vi "Begin.vi"(8 "error in":errorcluster) -> (0 "error out":errorcluster)   [LabVIEW 2015]
doc: "Called before other user functions, this VI is expected to open initial I/O refnums, load in file data, and do all program initialization. Notice that the <B>error out</B> terminal is simply used for data flow. Wiring it to other structures or subVIs ensures that this VI runs first."
uses:
  <vilib>/Rock Robotics/WPI/DriverStation/WPI_DriverStationRobotMode2.ctl
  <vilib>/Rock Robotics/WPI/Joystick/WPI_JoystickDeviceEnum.ctl
  <vilib>/Rock Robotics/SystemInterfaces/DIO/FPGA_DIOPWMChannel.ctl
  Robot Global Data.vi
  <vilib>/Rock Robotics/Network Tables/NT Write String Array.vi
  <vilib>/Rock Robotics/WPI/MotorControl/WPI_MotorControlOpen Talon.vi
  <vilib>/Rock Robotics/WPI/MotorControl/WPI_MotorControlOpen Victor.vi
  <vilib>/Rock Robotics/WPI/RobotDrive/WPI_RobotDriveOpen4MotorWithTalon.vi
  SubSystems/References/Refnums.vi
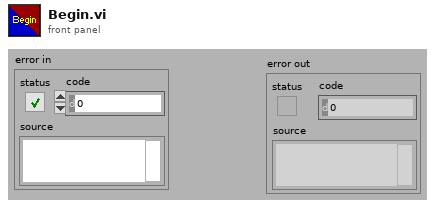
[diagram p1: front panel]
types:
  T1 = typedef "FPGA_DIOPWMChannel.ctl" = enum8{"PWM 0", "PWM 1", "PWM 2", "PWM 3", "PWM 4", "PWM 5", "PWM 6", "PWM 7", "PWM 8", "PWM 9", "PWM MXP 0", "PWM MXP 1", "PWM MXP 2", "PWM MXP 3", "PWM MXP 4", "PWM MXP 5", "PWM MXP 6", "PWM MXP 7", "PWM MXP 8", "PWM MXP 9", "Invalid"}
  T2 = typedef "WPI_JoystickDeviceEnum.ctl" = enum16{"USB 0", "USB 1", "USB 2", "USB 3", "USB 4", "USB 5"}
  T3 = typedef "WPI_DriverStationRobotMode2.ctl" = enum16{"Autonomous Disabled", "Autonomous Enabled", "Teleop Disabled", "Teleop Enabled", "Disconnected", "Finish", "Test Disabled", "Test Enabled", "Emergency Stopped"}
  T4 = typedef "WPI_JoystickDevRef.ctl" = cluster{"Device":T2}
  T5 = typedef "WPI_MotorControlDeviceRef.ctl" = cluster{"DeviceStatus":errorcluster, "Type":T6, "PWM":cluster{"PWM Channel":T1, "DeadBand":T7}, "CAN":cluster{"Device Number":u8, "Control Mode":T8, "Semaphore":T9, "Max Vout":dbl, "TalonSRX Control Mode":T10}, "Invert":bool}
  T6 = typedef "WPI_MotorControlType.ctl" = enum16{"PWM", "CAN", "CANTalonSRX"}
  T7 = typedef "WPI_PWMDeadband.ctl" = cluster{"Name":string, "maxPositivePwm":i32, "minPositivePwm":i32, "centerPwm":i32, "maxNegativePwm":i32, "minNegativePwm":i32, "angularRange":u16}
  T8 = typedef "WPI_CANJaguar_ControlMode.ctl" = enum8{"Percent VBus", "Current", "Speed", "Position", "Voltage"}
  T9 = typedef "Semaphore RefNum" = refnum<k1>
  T10 = typedef "WPI_CANTalonSRX_APIControlMode.ctl" = enum8{"Percent VBus", "Speed", "Position", "Slave", "Unchanged / Invalid", "Voltage Compensation", "Current", "Motion Profile"}
  T11 = typedef "WPI_RobotDriveDevRef.ctl" = cluster{"DevStatus":errorcluster, "Motors[]":T5[], "Square Inputs":bool, "Max Output":dbl}
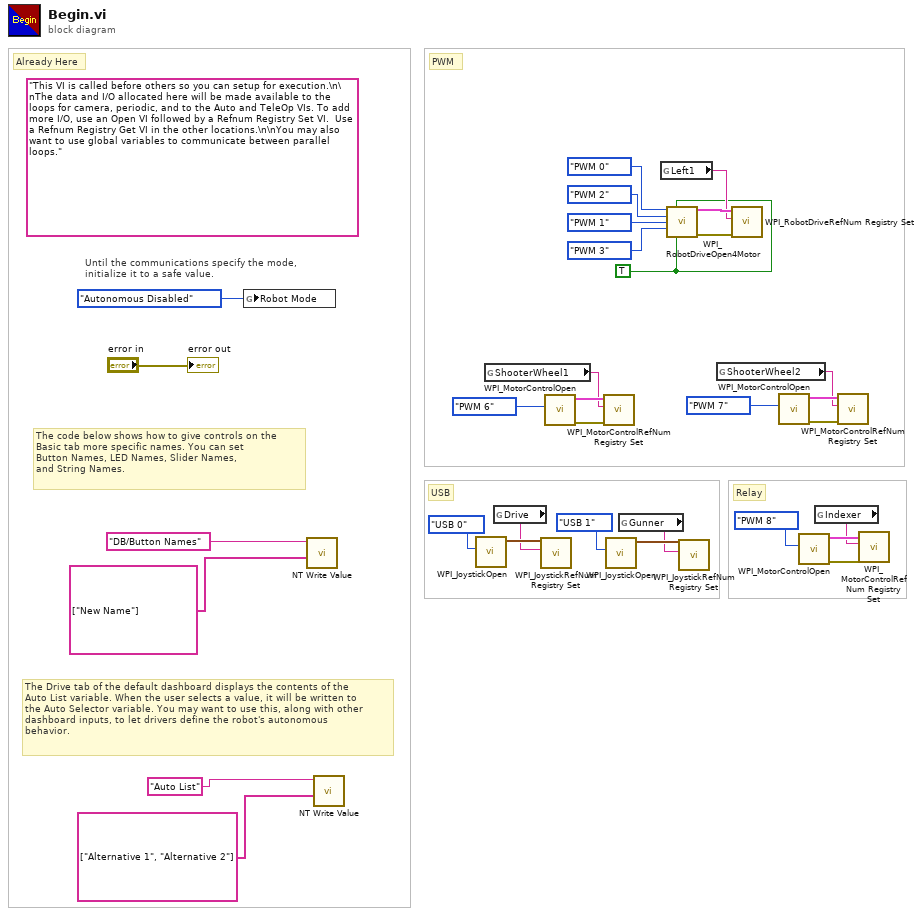
[diagram p0: block diagram]
diagram:
  w5 = TRUE ("Left Motor Inverted")
  (unwired) "This VI is called before others so you can setup for execution.\n\nThe data and I/O allocated here will be made available to the loops for camera, periodic, and to the Auto and TeleOp VIs. To add more I/O, use an Open VI followed by a Refnum Registry Set VI.  Use a Refnum Registry Get VI in the other locations.\n\nYou may also want to use global variables to communicate between parallel loops."
  # "PWM"
  # "Already Here"
  # "USB"
  # "Relay"
  # "The Drive tab of the default dashboard displays the contents of the\nAuto List variable. When the user selects a value, it will be written to\nthe Auto Selector variable. You may want to use this, along with other\ndashboard inputs, to let drivers define the robot's autonomous\nbehavior."
  # "The code below shows how to give controls on the\nBasic tab more specific names. You can set\nButton Names, LED Names, Slider Names,\nand String Names."
  # "Until the communications specify the mode,\ninitialize it to a safe value."
  n1 = global write "Robot Global Data.vi" "Robot Mode"(WPI_DriverStationRobotMode2."Autonomous Disabled" ("Robot Mode")) -> ()
  n2 = call-poly <vilib>:"NT Write Value.vi"("String Array"=string[] ["New Name"], "Name"="DB/Button Names") -> ()  [unwired: 9 in, 1 out]
  n3 = call-poly <vilib>:"NT Write Value.vi"("String Array"=string[] ["Alternative 1", "Alternative 2"], "Name"="Auto List") -> ()  [unwired: 9 in, 1 out]
  n4 = call <vilib>:"WPI_JoystickOpen.vi"("JoystickDevice"=WPI_JoystickDeviceEnum."USB 0") -> ("JoystickDevRef"=w26:T4)  [unwired: 10 in]
  n5 = global read "Refnums.vi" "ShooterWheel1"() -> (w13:string)
  n6 = global read "Refnums.vi" "Drive"() -> (w24:string)
  n7 = call <vilib>:"WPI_JoystickRefNum Registry Set.vi"("refnum name"=w24, "JoystickDevRef"=w26) -> ()  [unwired: 8 in, 2 out]
  n8 = call-poly <vilib>:"WPI_MotorControlOpen.vi"("PWM Channel"=FPGA_DIOPWMChannel."PWM 6") -> ("error out"=w15:errorcluster, "MotorControlDeviceRef"=w14:T5)  [unwired: 9 in]
  n9 = call <vilib>:"WPI_MotorControlRefNum Registry Set.vi"("error in (no error)"=w15, "refnum name"=w13, "MotorControlDevRef"=w14) -> ()  [unwired: 7 in, 2 out]
  n10 = call <vilib>:"WPI_JoystickOpen.vi"("JoystickDevice"=WPI_JoystickDeviceEnum."USB 1") -> ("JoystickDevRef"=w25:T4)  [unwired: 10 in]
  n11 = global read "Refnums.vi" "Gunner"() -> (w23:string)
  n12 = global read "Refnums.vi" "Left1"() -> (w6:string)
  n13 = call-poly <vilib>:"WPI_RobotDriveOpen4Motor.vi"("Rear Left Motor"=FPGA_DIOPWMChannel."PWM 0" ("Right Motor"), "Rear Left Motor Inverted"=w5, "Rear Right Motor"=FPGA_DIOPWMChannel."PWM 2" ("Left Motor"), "Front Left Motor"=FPGA_DIOPWMChannel."PWM 1" ("Left Motor"), "Front Right Motor"=FPGA_DIOPWMChannel."PWM 3" ("Left Motor"), "Front Left Motor Inverted"=w5) -> ("RobotDriveDevRef"=w8:T11, "error out"=w7:errorcluster)  [unwired: 8 in]
  n14 = call <vilib>:"WPI_JoystickRefNum Registry Set.vi"("refnum name"=w23, "JoystickDevRef"=w25) -> ()  [unwired: 8 in, 2 out]
  n15 = global read "Refnums.vi" "ShooterWheel2"() -> (w16:string)
  n16 = call <vilib>:"WPI_RobotDriveRefNum Registry Set.vi"("error in (no error)"=w7, "refnum name"=w6, "RobotDriveDevRef"=w8) -> ()  [unwired: 7 in, 2 out]
  n17 = call-poly <vilib>:"WPI_MotorControlOpen.vi"("PWM Channel"=FPGA_DIOPWMChannel."PWM 7") -> ("error out"=w18:errorcluster, "MotorControlDeviceRef"=w17:T5)  [unwired: 9 in]
  n18 = call-poly <vilib>:"WPI_MotorControlOpen.vi"("PWM Channel"=FPGA_DIOPWMChannel."PWM 8") -> ("error out"=w11:errorcluster, "MotorControlDeviceRef"=w10:T5)  [unwired: 9 in]
  n19 = global read "Refnums.vi" "Indexer"() -> (w9:string)
  n20 = call <vilib>:"WPI_MotorControlRefNum Registry Set.vi"("error in (no error)"=w18, "refnum name"=w16, "MotorControlDevRef"=w17) -> ()  [unwired: 7 in, 2 out]
  n21 = call <vilib>:"WPI_MotorControlRefNum Registry Set.vi"("error in (no error)"=w11, "refnum name"=w9, "MotorControlDevRef"=w10) -> ()  [unwired: 7 in, 2 out]
  "error out" <- "error in"
